vi "Get Server CRC Support.vi"(8 "error in":errorcluster, 11 "Block Upload Initiate Transfer in":refnum<class "Block Upload Initiate Transfer.lvclass">) -> (0 "error out":errorcluster, 2 "Server CRC Support":bool, 3 "Block Upload Initiate Transfer out":refnum<class "Block Upload Initiate Transfer.lvclass">)   [LabVIEW 2020, in "CANopen.lvlib" / "SDO Manager.lvlib" / "Block Upload Initiate Transfer.lvclass"]
uses:
  Block Upload Initiate Transfer.lvclass
  Block Upload Initiate Transfer.lvclass/Block Upload Initiate Transfer.ctl
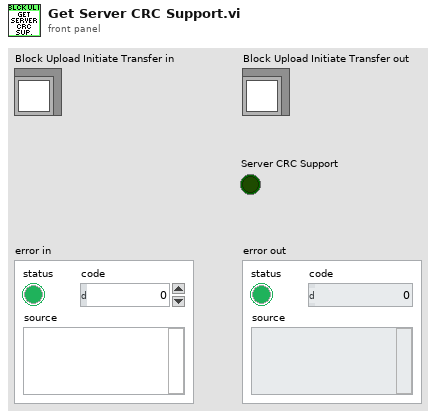
[diagram p1: front panel]
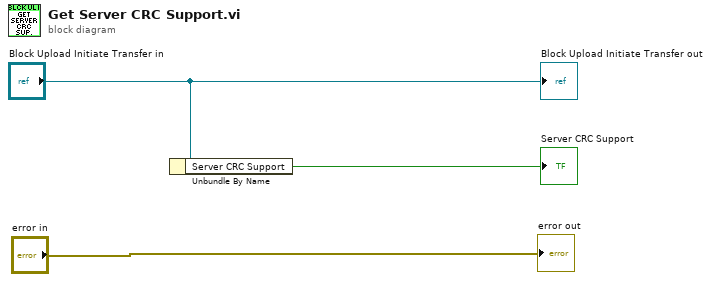
[diagram p0: block diagram]
diagram:
  n1 = Unbundle By Name("Block Upload Initiate Transfer in") -> ("Server CRC Support"=→"Server CRC Support":bool)
  "error out" <- "error in"
  "Block Upload Initiate Transfer out" <- "Block Upload Initiate Transfer in"
